vi "Single Class_Multiple_State_External_4.vi"(0 "HSMO#4":refnum<class "Hyper_State_Machine.lvclass">, 1 "State_Interval_Time(s)":dbl=0.001 min=0.0 max=86400.0 format="%#_13p", 2 "Time Target (s)":dbl=30.0 format="%#_13g", 3 "System_Delay(s)":dbl=0.01 min=0.0 max=86400.0 format="%#_13p") -> ()   [LabVIEW 2021]
uses:
  C:/Program Files (x86)/Hyper State Machine Framework/SSW_Hyper_State_Machine.lvlibp/State_Machine_Class/Main_State_Machine/Hyper_State_Machine.lvclass
  C:/Program Files (x86)/Hyper State Machine Framework/SSW_Hyper_State_Machine.lvlibp/State_Machine_Class/State_Machine_Module.llb/State Machine[].ctl
  C:/Program Files (x86)/Hyper State Machine Framework/SSW_Hyper_State_Machine.lvlibp/State_Machine_Class/State_Machine_Module.llb/Iterval.ctl
  C:/Program Files (x86)/Hyper State Machine Framework/SSW_Hyper_State_Machine.lvlibp/State_Machine_Class/State_Machine_Module.llb/Lock_Unlock.ctl
  C:/Program Files (x86)/Hyper State Machine Framework/SSW_Hyper_State_Machine.lvlibp
panel:
  out "Implementation Class":string
  out "Current State":string
  out "Show_Stop_Button":bool=TRUE
  in  "Unlock":bool
  in  "Reset":bool
  in  "lock All":bool
  in  "Stop":bool
  out "Timing":dbl
  out "Lock":bool
  # "HSMO#4"
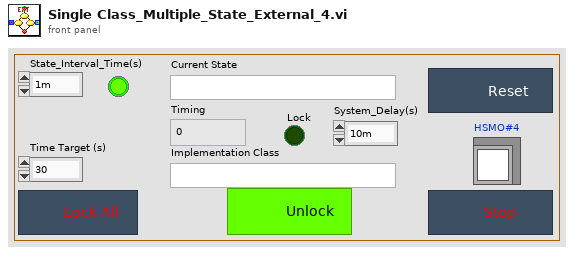
[diagram p1: front panel]
types:
  T1 = typedef "SSW_Hyper_State_Machine.lvlibp/State Machine[].ctl" = cluster{"Command":string, "Data":variant}[]
  T2 = typedef "SSW_Hyper_State_Machine.lvlibp/Lock_Unlock.ctl" = cluster{"Action_Mode (Get)":enum16{"Set", "Get"}, "Action_Set (False)":bool, "State_In (Wait)":string}
  T3 = typedef "SSW_Hyper_State_Machine.lvlibp/Iterval.ctl" = cluster{"Delay(s)":dbl, "State (Interval_Delay)":string}
  T4 = typedef "SSW_Hyper_State_Machine.lvlibp/State Machine.ctl" = cluster{"Command":string, "Data":variant}
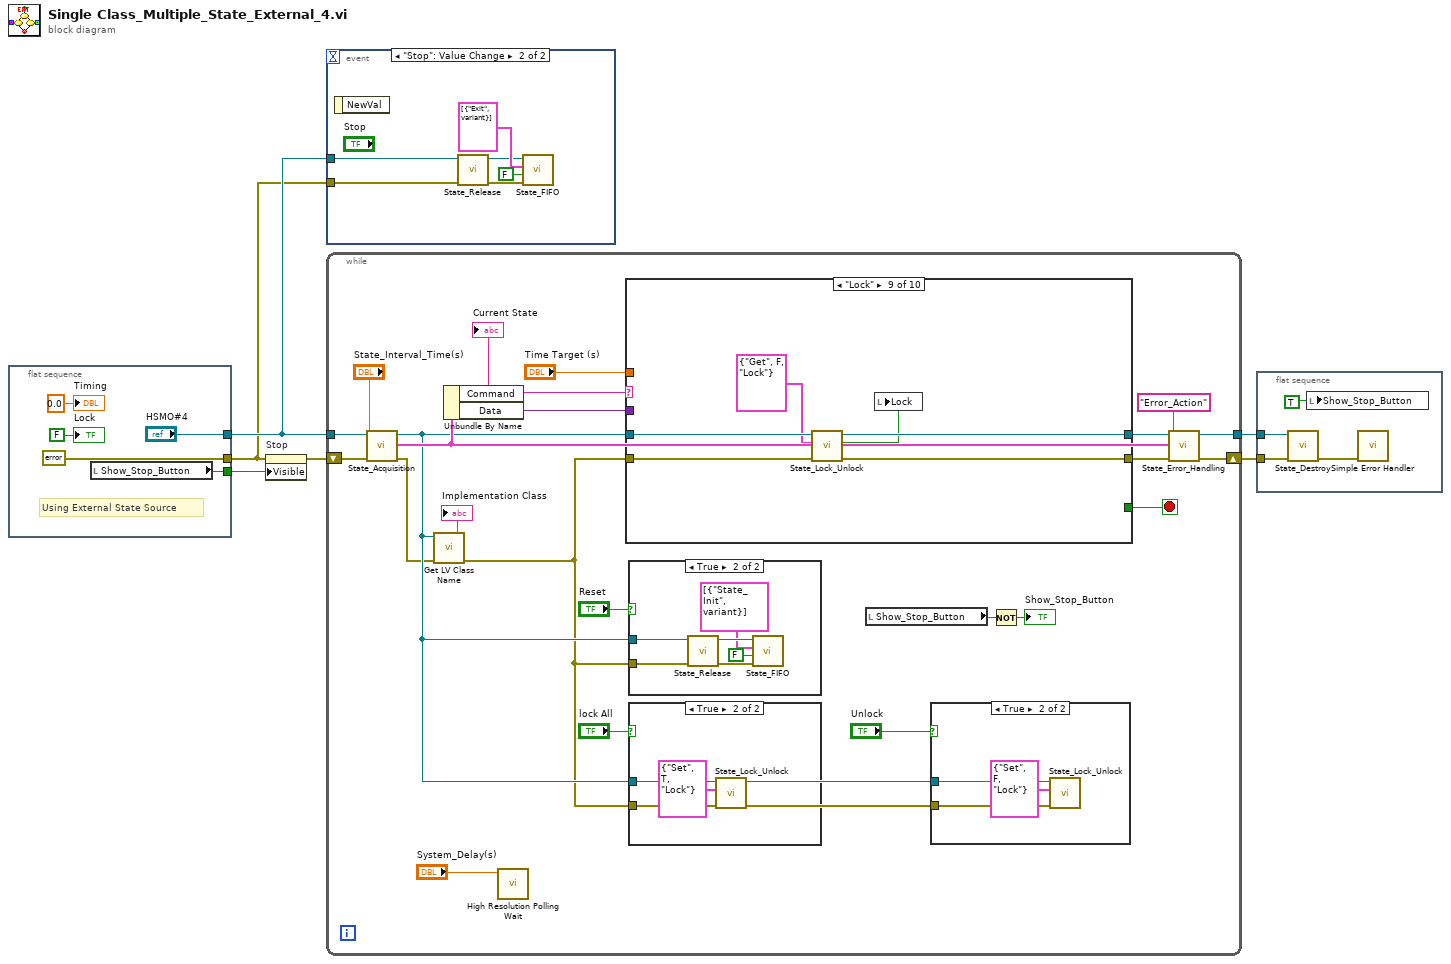
[diagram p0: block diagram]
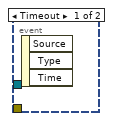
[diagram p2: hidden frame]
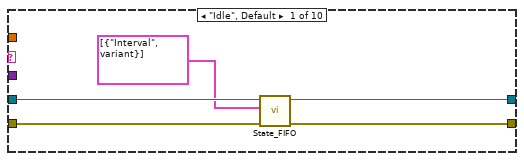
[diagram p6: hidden frame]
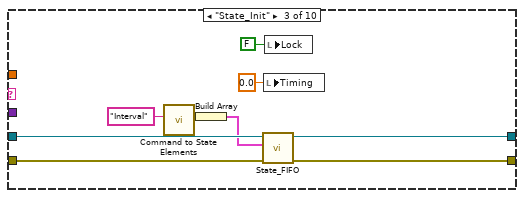
[diagram p8: hidden frame]
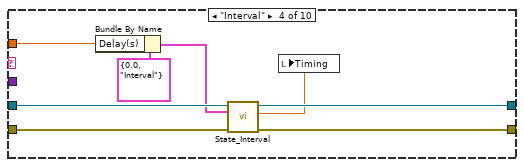
[diagram p9: hidden frame]
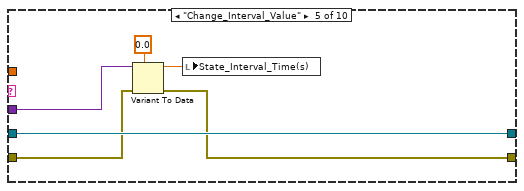
[diagram p10: hidden frame]
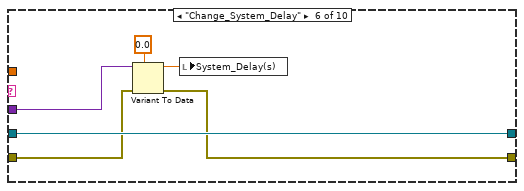
[diagram p11: hidden frame]
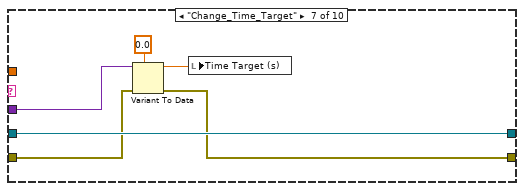
[diagram p12: hidden frame]
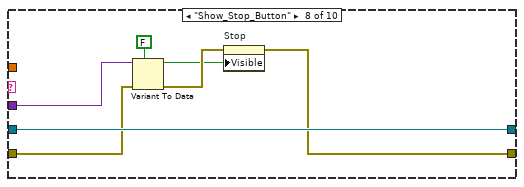
[diagram p13: hidden frame]
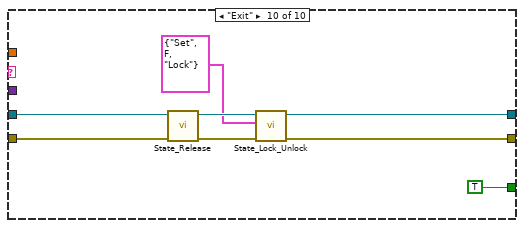
[diagram p14: hidden frame]
diagram:
  n1 = flat-sequence {
    tunnel: ["HSMO#4"] -> w3
    tunnel: [errorcluster {"status"=FALSE, "code"=0, "source"=""} ("error out")] -> w2
    tunnel: [w7] -> w1
    frame #0 {
      # "Using External State Source"
      n2 = local read "Show_Stop_Button"() -> (w7:bool)
      "Lock" <- FALSE ("Lock")
      "Timing" <- 0.0 ("Timing")
    }
  }
  n3 = property on="Stop" class="Bool"(error in=w2, "Visible"=w1) -> (error out=w4:errorcluster)  [unwired: 1 in, 1 out]
  n4 = event shown="[1] \"Stop\": Value Change" {
    selector: _ -> [_ _]
    dyn-events: _ -> [_ _]
    timeout: _ -> [_ _]
    tunnel: w3 -> [_ w17]
    tunnel: w2 -> [_ w16]
    event Timeout {
      n5 = event-data() -> ()  [unwired: 1 in, 3 out]
    }
    event "Stop": Value Change {
      n6 = event-data() -> ()  [unwired: 1 in, 1 out]
      n7 = call-dynamic "State_Release.vi"("error in (no error)"=w16, "State_Machine_Class in"=w17) -> ("error out"=w13:errorcluster, "State_Machine_Class out"=w12:refnum<class "Hyper_State_Machine.lvclass">)  [unwired: 8 in]
      n8 = call-dynamic "State_FIFO.vi"("error in (no error)"=w13, "State_Interval(Enable)"=FALSE, "State Machine[]"=T1 [{"Command"="Exit", "Data"=variant}], "State_Machine_Class in"=w12) -> ()  [unwired: 6 in, 2 out]
    }
  }
  n9 = while {
    tunnel: w3 -> [w40]
    tunnel: [w37] -> w6
    shift-right: [w36] -> w5
    shift-left: w4 -> [w39]
    stop <- w38 stop-if-true
    n10 = call-dynamic "State_Acquisition.vi"("error in (no error)"=w39, "State_Interval_Time(s)"="State_Interval_Time(s)", "Main_Machine_State_Class in"=w40) -> ("error out"=w20:errorcluster, "State"=w27:T4, "Main_Machine_State_Class out"=w21:refnum<class "Hyper_State_Machine.lvclass">)  [unwired: 2 in, 4 out]
    n11 = call <vilib>:"Get LV Class Name.vi"("error in (no error)"=w20, "object"=w21) -> ("error out"=w18:errorcluster, "class name"=→"Implementation Class":string)  [unwired: 8 in]
    n12 = Unbundle By Name(w27) -> ("Command"=w23:string, "Data"=w28:variant)
    "Current State" <- w23
    n13 = call <vilib>:"High Resolution Polling Wait.vi"("seconds to wait"="System_Delay(s)") -> ()  [unwired: 10 in, 1 out]
    n14 = case shown="\"Lock\"" w23 {
      tunnel: w28 -> [_ _ _ _ w81 w87 w93 w100 _ _]
      tunnel: w21 -> [w57 w59 w68 w74 w82 w88 w94 w101 w107 w114]
      tunnel: w18 -> [w56 w58 w66 w73 w80 w86 w92 w99 w106 w113]
      tunnel: [w55 w59 w67 w71 w82 w88 w94 w101 w105 w110] -> w25
      tunnel: [w54 w58 w65 w70 w79 w85 w91 w95 w104 w109] -> w24
      tunnel: [_ _ _ _ _ _ _ _ _ TRUE] -> w38
      tunnel: "Time Target (s)" -> [_ _ _ w76 _ _ _ _ _ _]
      frame "Idle", Default {
        n15 = call-dynamic "State_FIFO.vi"("error in (no error)"=w56, "State Machine[]"=T1 [{"Command"="Interval", "Data"=variant}], "State_Machine_Class in"=w57) -> ("error out"=w54:errorcluster, "State_Machine_Class out"=w55:refnum<class "Hyper_State_Machine.lvclass">)  [unwired: 7 in]
      }
      frame "State_Interval" {
        # "Execute Every Define of State Interval Time"
      }
      frame "State_Init" {
        n16 = call "Command to State Elements.vi"("Command"="Interval") -> ("Command to State Elements"=w63:T4)  [unwired: 10 in]
        n17 = Build Array(w63) -> (w62:T4[])
        n18 = call-dynamic "State_FIFO.vi"("error in (no error)"=w66, "State Machine[]"=w62, "State_Machine_Class in"=w68) -> ("error out"=w65:errorcluster, "State_Machine_Class out"=w67:refnum<class "Hyper_State_Machine.lvclass">)  [unwired: 7 in]
        n19 = local write "Timing"(0.0 ("Timing")) -> ()
        n20 = local write "Lock"(FALSE ("Lock")) -> ()
      }
      frame "Interval" {
        n21 = Bundle By Name(cluster=T3 {"Delay(s)"=0.0, "State (Interval_Delay)"="Interval"} ("Parameter"), "Delay(s)"=w76) -> (w72:T3)
        n22 = call-dynamic "State_Interval.vi"("error in (no error)"=w73, "Parameter"=w72, "State_Machine_Class in"=w74) -> ("error out"=w70:errorcluster, "Elapsed Time(s)"=w69:dbl, "State_Machine_Class out"=w71:refnum<class "Hyper_State_Machine.lvclass">)  [unwired: 6 in]
        n23 = local write "Timing"(w69) -> ()
      }
      frame "Change_Interval_Value" {
        n24 = Variant To Data(error in=w80, type=0.0 ("Time Target (s)"), Variant=w81) -> (data=w77:dbl, error out=w79:errorcluster)
        n25 = local write "State_Interval_Time(s)"(w77) -> ()
      }
      frame "Change_System_Delay" {
        n26 = Variant To Data(error in=w86, type=0.0 ("Time Target (s)"), Variant=w87) -> (data=w83:dbl, error out=w85:errorcluster)
        n27 = local write "System_Delay(s)"(w83) -> ()
      }
      frame "Change_Time_Target" {
        n28 = Variant To Data(error in=w92, type=0.0 ("Time Target (s)"), Variant=w93) -> (data=w89:dbl, error out=w91:errorcluster)
        n29 = local write "Time Target (s)"(w89) -> ()
      }
      frame "Show_Stop_Button" {
        n30 = Variant To Data(error in=w99, type=FALSE, Variant=w100) -> (data=w96:bool, error out=w97:errorcluster)
        n31 = property on="Stop" class="Bool"(error in=w97, "Visible"=w96) -> (error out=w95:errorcluster)  [unwired: 1 in, 1 out]
      }
      frame "Lock" {
        n32 = call-dynamic "State_Lock_Unlock.vi"("error in (no error)"=w106, "Parameter"=T2 {"Action_Mode (Get)"=enum."Get", "Action_Set (False)"=FALSE, "State_In (Wait)"="Lock"}, "State_Machine_Class in"=w107) -> ("error out"=w104:errorcluster, "Action_Get"=w102:bool, "State_Machine_Class out"=w105:refnum<class "Hyper_State_Machine.lvclass">)  [unwired: 6 in]
        n33 = local write "Lock"(w102) -> ()
      }
      frame "Exit" {
        n34 = call-dynamic "State_Release.vi"("error in (no error)"=w113, "State_Machine_Class in"=w114) -> ("error out"=w111:errorcluster, "State_Machine_Class out"=w112:refnum<class "Hyper_State_Machine.lvclass">)  [unwired: 8 in]
        n35 = call-dynamic "State_Lock_Unlock.vi"("error in (no error)"=w111, "Parameter"=T2 {"Action_Mode (Get)"=enum."Set", "Action_Set (False)"=FALSE, "State_In (Wait)"="Lock"}, "State_Machine_Class in"=w112) -> ("error out"=w109:errorcluster, "State_Machine_Class out"=w110:refnum<class "Hyper_State_Machine.lvclass">)  [unwired: 6 in, 1 out]
      }
    }
    n36 = case shown="True" "Reset" {
      tunnel: w21 -> [_ w52]
      tunnel: w18 -> [_ w48]
      frame False {
      }
      frame True {
        n37 = call-dynamic "State_Release.vi"("error in (no error)"=w48, "State_Machine_Class in"=w52) -> ("error out"=w50:errorcluster, "State_Machine_Class out"=w51:refnum<class "Hyper_State_Machine.lvclass">)  [unwired: 8 in]
        n38 = call-dynamic "State_FIFO.vi"("error in (no error)"=w50, "State_Interval(Enable)"=FALSE, "State Machine[]"=T1 [{"Command"="State_Init", "Data"=variant}], "State_Machine_Class in"=w51) -> ()  [unwired: 6 in, 2 out]
      }
    }
    n39 = case shown="True" "lock All" {
      tunnel: w21 -> [_ w46]
      tunnel: w18 -> [_ w45]
      frame False {
      }
      frame True {
        n40 = call-dynamic "State_Lock_Unlock.vi"("error in (no error)"=w45, "Parameter"=T2 {"Action_Mode (Get)"=enum."Set", "Action_Set (False)"=TRUE, "State_In (Wait)"="Lock"}, "State_Machine_Class in"=w46) -> ()  [unwired: 6 in, 3 out]
      }
    }
    n41 = local read "Show_Stop_Button"() -> (w30:bool)
    n42 = case shown="True" "Unlock" {
      tunnel: w21 -> [_ w42]
      tunnel: w18 -> [_ w43]
      frame False {
      }
      frame True {
        n43 = call-dynamic "State_Lock_Unlock.vi"("error in (no error)"=w43, "Parameter"=T2 {"Action_Mode (Get)"=enum."Set", "Action_Set (False)"=FALSE, "State_In (Wait)"="Lock"}, "State_Machine_Class in"=w42) -> ()  [unwired: 6 in, 3 out]
      }
    }
    n44 = Not(x=w30) -> (.not. x?=→"Show_Stop_Button":bool)
    n45 = call-dynamic "State_Error_Handling.vi"("error in (no error)"=w24, "Reply_State_Name"="Error_Action", "Handling_State(State_Acquisition)"=w27, "State_Machine_Class in"=w25) -> ("error out"=w36:errorcluster, "State_Machine_Class out"=w37:refnum<class "Hyper_State_Machine.lvclass">)  [unwired: 6 in]
  }
  n46 = flat-sequence {
    tunnel: w6 -> [w118]
    tunnel: w5 -> [w117]
    frame #0 {
      n47 = call-dynamic "State_Destroy.vi"("error in (no error)"=w117, "State_Machine_Class in"=w118) -> ("error out"=w119:errorcluster)  [unwired: 9 in]
      n48 = local write "Show_Stop_Button"(TRUE ("Show_Stop_Button")) -> ()
      n49 = call <vilib>:"Simple Error Handler.vi"("error in (no error)"=w119) -> ()  [unwired: 4 in, 5 out]
    }
  }
